vi "Move waveplate.vi"(8 "error in (no error)":errorcluster, 9 "Angle":dbl, 10 "Axis in":i32, 11 "VISA Refnum in":refnum<visa-resource-name>) -> (0 "error out":errorcluster, 1 "WP Error":bool, 2 "Current position (units)":dbl, 3 "VISA Refnum out":refnum<visa-resource-name>)   [LabVIEW 2013]
panel:
  in  "Delay":u32
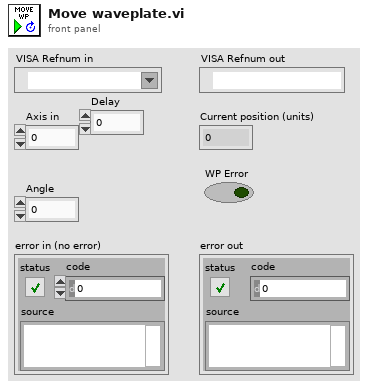
[diagram p1: front panel]
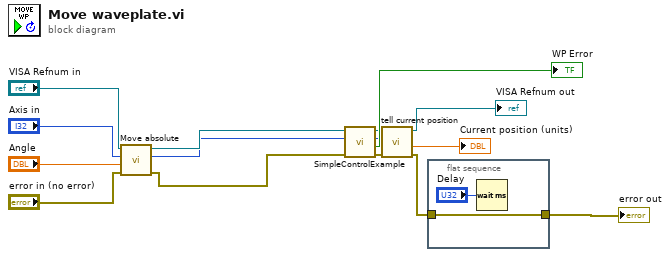
[diagram p0: block diagram]
diagram:
  n1 = call "Move absolute.vi"("error in"="error in (no error)", "New target position (units)"="Angle", "Axis in"="Axis in", "VISA Handle in"="VISA Refnum in") -> ("error out"=w1:errorcluster, "Axis out"=w7:i32, "VISA Handle out"=w8:refnum<visa-resource-name>)  [unwired: 2 in, 1 out]
  n2 = call "SimpleControlExample.vi"("error in"=w1, "Axis in"=w7, "VISA Handle in"=w8) -> ("error out"=w9:errorcluster, "WP Error"=→"WP Error":bool, "Axis out"=w10:i32, "VISA Handle out"=w11:refnum<visa-resource-name>)  [unwired: 2 in, 1 out]
  n3 = call "tell current position.vi"("error in"=w9, "Axis in"=w10, "VISA Handle in"=w11) -> ("error out"=w2:errorcluster, "Current position (units)"=→"Current position (units)":dbl, "VISA Handle out"=→"VISA Refnum out":refnum<visa-resource-name>)  [unwired: 2 in, 2 out]
  n4 = flat-sequence {
    tunnel: [w17] -> w3
    tunnel: w2 -> [w17]
    frame #0 {
      n5 = Wait (ms)(milliseconds to wait="Delay") -> ()  [unwired: 1 out]
    }
  }
  "error out" <- w3
